vi "IPI_SaveImage.vi"(6 "ccdorlaser":string, 7 "File Path":path=path "C:/GapAndFlatnessMesaure/Source Code/Image", 8 "error in (no error)":errorcluster, 9 "Barcode":string, 10 "name":string, 11 "Image 2":T1(plugin-control)) -> (0 "error out":errorcluster, 3 "Image Out (duplicate)":T1)   [LabVIEW 2015]
uses:
  <vilib>/vision/Image Controls.llb/IMAQ Image.ctl
panel:
  out "路径":path
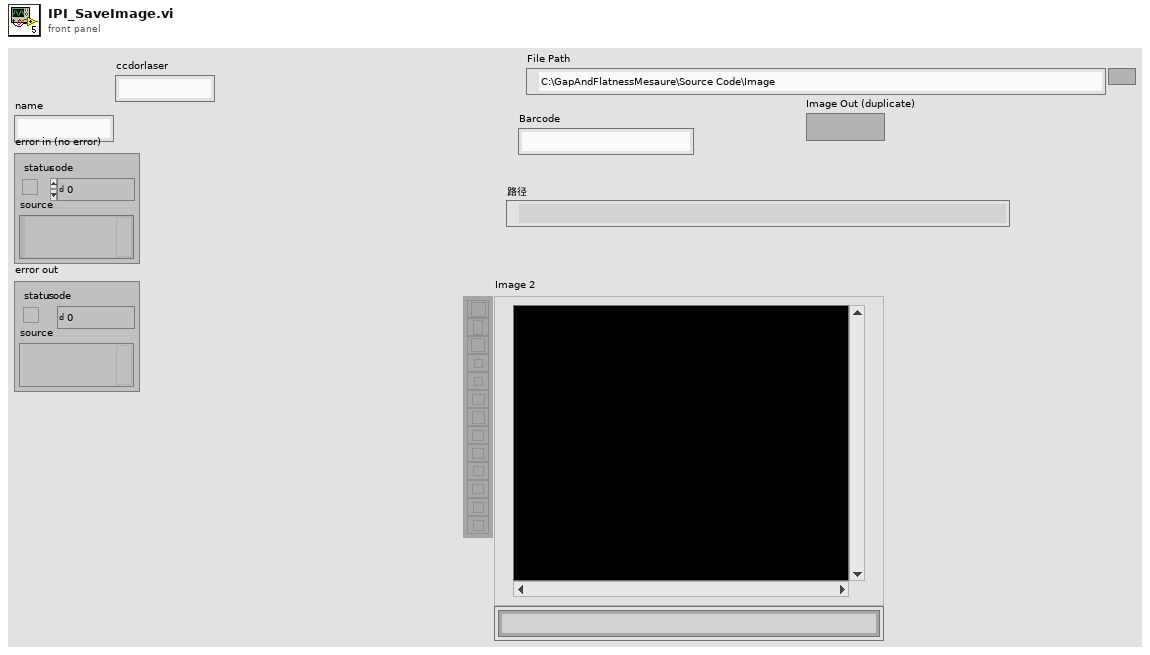
[diagram p1: front panel]
types:
  T1 = typedef "IMAQ Image.ctl" = refnum<image>
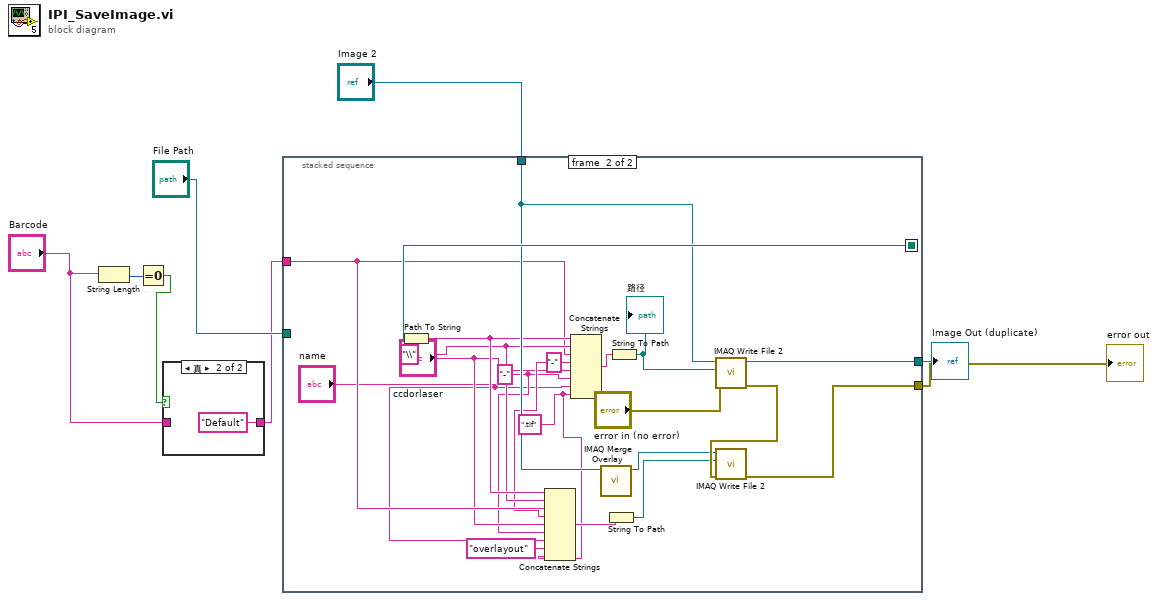
[diagram p0: block diagram]
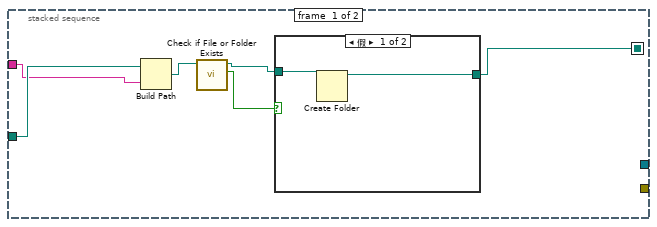
[diagram p3: hidden frame]
diagram:
  n1 = String Length(string="Barcode") -> (length=w6:i32)
  n2 = Equal To 0?(x=w6) -> (x = 0?=w5:bool)
  n3 = case shown="真" w5 {
    tunnel: "Barcode" -> [w9 _]
    tunnel: [w9 "Default" ("Barcode")] -> w3
    frame False {
    }
    frame True {
    }
  }
  n4 = stacked-sequence {
    seq-local: [w14 _] -> [_ w36]
    tunnel: "File Path" -> [w16 _]
    tunnel: [_ w32] -> w7
    tunnel: w3 -> [w15 w26]
    tunnel: [_ w35] -> w2
    tunnel: "Image 2" -> [_ w34]
    frame #0 {
      n5 = Build Path(base path=w16, name or relative path=w15) -> (appended path=w13:path)
      n6 = call <vilib>:"Check if File or Folder Exists.vi"("path"=w13) -> ("file or folder exists?"=w12:bool, "dup path"=w11:path)  [unwired: 8 in, 1 out]
      n7 = case shown="假" w12 {
        tunnel: w11 -> [w18 w19]
        tunnel: [w17 w19] -> w14
        frame False {
          n8 = Create Folder(path (use dialog)=w18) -> (created path=w17:path)  [unwired: 2 in, 2 out]
        }
        frame True {
        }
      }
    }
    frame #1 {
      w25 = "-" ("字符串")
      w23 = "-" ("字符串")
      w21 = ".tif" ("字符串")
      w27 = "\\" ("字符串")
      n9 = Path To String(path=w36) -> (string=w28:string)
      n10 = Concatenate Strings(w28, w27, w26, w25, "ccdorlaser", w23, "name", "overlayout" ("字符串"), w21) -> (w30:string)
      n11 = Concatenate Strings(w28, w27, w26, w25, "ccdorlaser", w23, "name", w21) -> (w39:string)
      n12 = call "IMAQ Merge Overlay"("Image Src"=w34) -> ("Image Dst Out"=w31:T1)  [unwired: 9 in, 1 out]
      n13 = String To Path(string=w30) -> (path=w29:path)
      n14 = String To Path(string=w39) -> (path=w38:path)
      "路径" <- w38
      n15 = call-poly "IMAQ Write File 2"("error in (no error)"="error in (no error)", "File Path"=w38, "Image"=w34) -> ("error out"=w33:errorcluster, "Image Out (duplicate)"=w35:T1)  [unwired: 7 in]
      n16 = call-poly "IMAQ Write File 2"("error in (no error)"=w33, "File Path"=w29, "Image"=w31) -> ("error out"=w32:errorcluster)  [unwired: 7 in, 1 out]
    }
  }
  "error out" <- w7
  "Image Out (duplicate)" <- w2
